vi "실습2-3수식노드사용.vi"() -> ()   [LabVIEW 2014]
panel:
  out "C":dbl format="%#_15f"
  in  "B":dbl
  out "웨이브폼 그래프":dbl[](graph)
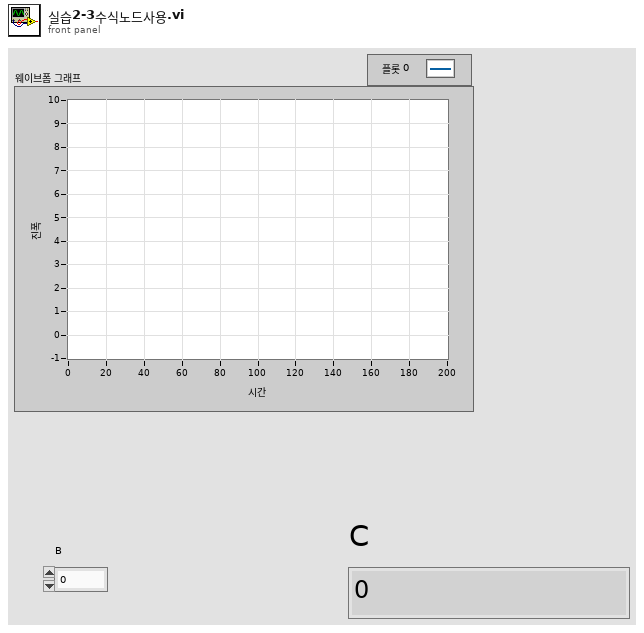
[diagram p1: front panel]
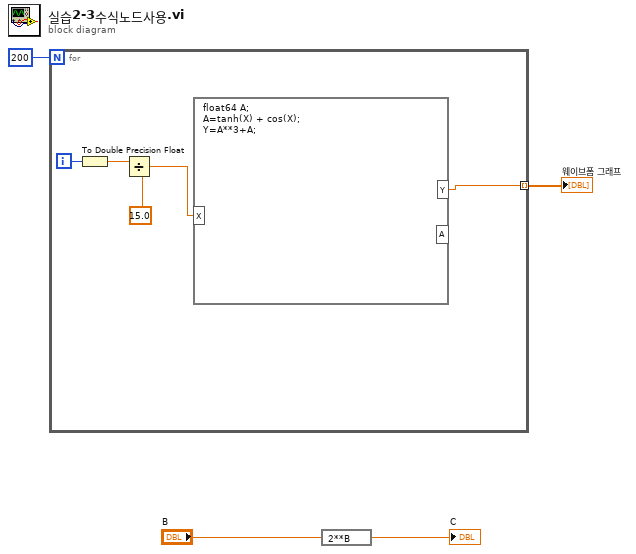
[diagram p0: block diagram]
diagram:
  n1 = for {
    N: 200 -> [_]
    tunnel: [w5] -> w3 mode=indexing
    i -> [w9]
    n2 = To Double Precision Float(number=w9) -> (double precision float=w8:dbl)
    n3 = Divide(x=w8, y=15.0) -> (x/y=w6:dbl)
    n4 = formula code="float64 A;\nA=tanh(X) + cos(X);\nY=A**3+A;"("X"=w6) -> ("Y"=w5:dbl)  [unwired: 1 out]
  }
  "웨이브폼 그래프" <- w3
  n5 = expression code="2**B"("B") -> (→"C":dbl)
